vi "Teleop.vi"(10 "Match Info":T1={"Autonomous Elapsed Seconds"=0.0, "TeleOp Elapsed Seconds"=0.0, "Disabled Elapsed Seconds"=0.0, "Visited Autonomous"=FALSE, "Visited TeleOp"=FALSE, "Visited Disabled"=FALSE, "Autonomous Settings"={"Autonomous Style"=enum."Independent", "VI Refnum"=refnum}}, 11 "Call Context":T2) -> ()   [LabVIEW 2013]
doc: "This VI is called for each TeleOp packet received from the DS where the robot is not disabled. It is often used to read from the joysticks and update I/O or to update setpoints for timed control loops. It should complete and return within 20 milliseconds or it may miss DS packets."
uses:
  Specials/Global Data.vi
  <vilib>/Rock Robotics/WPI/DriverStation/WPI_DriverStationMatch Info.ctl
  <vilib>/Rock Robotics/WPI/DriverStation/WPI_DriverStationDerivedRobotMode.ctl
panel:
  in  "Xbox Controller?":bool
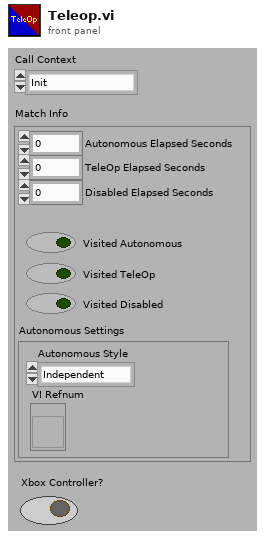
[diagram p1: front panel]
types:
  T1 = typedef "WPI_DriverStationMatch Info.ctl" = cluster{"Autonomous Elapsed Seconds":dbl, "TeleOp Elapsed Seconds":dbl, "Disabled Elapsed Seconds":dbl, "Visited Autonomous":bool, "Visited TeleOp":bool, "Visited Disabled":bool, "Autonomous Settings":cluster{"Autonomous Style":enum16{"Iterative", "Independent"}, "VI Refnum":refnum<vi>}}
  T2 = typedef "WPI_DriverStationDerivedRobotMode.ctl" = enum16{"Init", "Execute", "Stop"}
  T3 = typedef "WPI_JoystickDevRef.ctl" = cluster{"Device":T4}
  T4 = typedef "WPI_JoystickDeviceEnum.ctl" = enum16{"USB 1", "USB 2", "USB 3", "USB 4", "Kinect 1", "Kinect 2"}
  T5 = cluster{"axis 1 (x)":dbl, "axis 2 (y)":dbl, "axis 3 (throttle)":dbl, "axis 4":dbl, "axis 5":dbl, "axis 6":dbl}
  T6 = typedef "WPI_JoystickButtonState.ctl" = cluster{"Button 1":bool, "Button 2":bool, "Button 3":bool, "Button 4":bool, "Button 5":bool, "Button 6":bool, "Button 7":bool, "Button 8":bool, "Button 9":bool, "Button 10":bool, "Button 11":bool, "Button 12":bool}
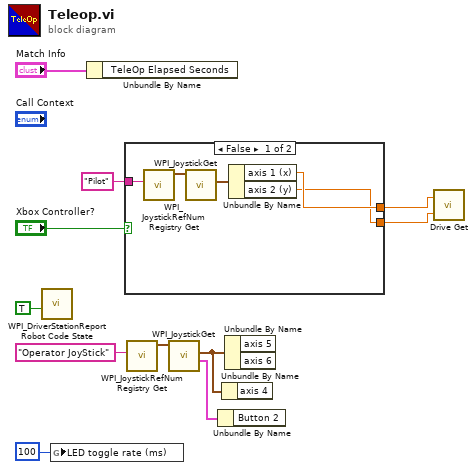
[diagram p0: block diagram]
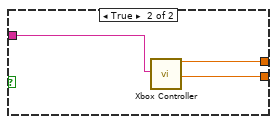
[diagram p2: hidden frame]
diagram:
  n1 = call <vilib>:"WPI_DriverStationReport Robot Code State.vi"("TeleOp"=TRUE ("Autonomous")) -> ()  [unwired: 10 in, 1 out]
  n2 = global write "Global Data.vi" "LED toggle rate (ms)"(u32 100 ("LED ms toggle rate")) -> ()
  n3 = Unbundle By Name("Match Info") -> ()  [unwired: 1 out]
  n4 = case shown="False" "Xbox Controller?" {
    tunnel: "Pilot" ("refnum name") -> [w15 w19]
    tunnel: [w13 w18] -> w2
    tunnel: [w12 w17] -> w1
    frame False {
      n5 = call <vilib>:"WPI_JoystickRefNum Registry Get.vi"("refnum name"=w15) -> ("JoystickDevRef"=w16:T3)  [unwired: 9 in, 1 out]
      n6 = call <vilib>:"WPI_JoystickGet.vi"("JoystickDevRef"=w16) -> ("Axes"=w14:T5)  [unwired: 4 in, 2 out]
      n7 = Unbundle By Name(w14) -> ("axis 1 (x)"=w13:dbl, "axis 2 (y)"=w12:dbl)
    }
    frame True {
      n8 = call "Xbox Controller.vi"("Joystick Name"=w19) -> ("Left Stick Y"=w18:dbl, "Right Stick Y"=w17:dbl)  [unwired: 3 in, 14 out]
    }
  }
  n9 = call <vilib>:"WPI_JoystickRefNum Registry Get.vi"("refnum name"="Operator JoyStick") -> ("JoystickDevRef"=w8:T3)  [unwired: 9 in, 1 out]
  n10 = call <vilib>:"WPI_JoystickGet.vi"("JoystickDevRef"=w8) -> ("Buttons"=w3:T6, "Axes"=w6:T5)  [unwired: 4 in, 1 out]
  n11 = Unbundle By Name(w3) -> ()  [unwired: 1 out]
  n12 = Unbundle By Name(w6) -> ()  [unwired: 1 out]
  n13 = Unbundle By Name(w6) -> ()  [unwired: 2 out]
  n14 = call "Drive Get.vi"("Y"=w1, "X"=w2) -> ()  [unwired: 1 in]
